vi "simple shutter control.vi"() -> ()   [LabVIEW 2016]
panel:
  in  "?":bool[](array[boolean])=[FALSE, FALSE, FALSE]
  in  "stop":bool
  # "IR"
  # "Red"
  # "Green"
  # "Blue"
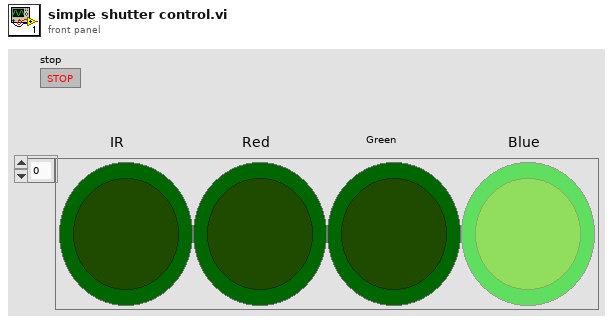
[diagram p1: front panel]
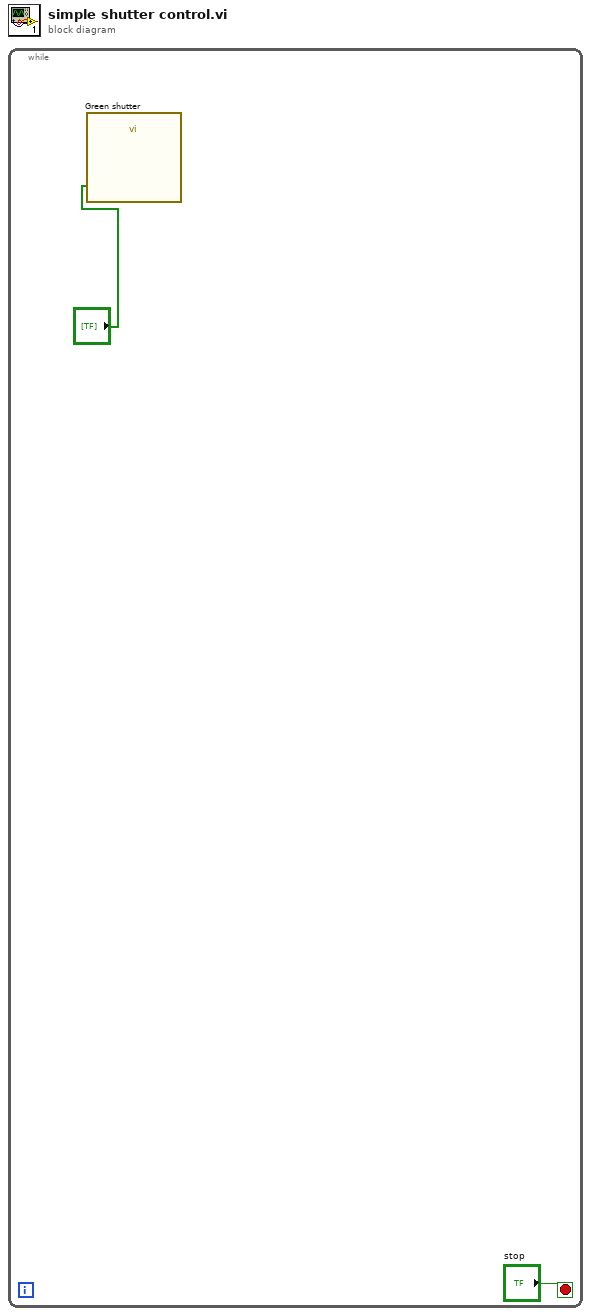
[diagram p0: block diagram]
diagram:
  n1 = while {
    stop <- "stop" stop-if-true
    n2 = call "Green shutter"("data"="?") -> ()  [unwired: 17 in, 2 out]
  }
